vi "BuildTestFromProjectItem_Library_SetsTestSuiteName.vi"() -> ()   [LabVIEW 2017, in "LVUnitTestBuilderTest.lvlib"]
uses:
  LVUnitTestBuilderTest.lvlib
  LVUnitTestBuilder/LVUnitTestBuilder.lvclass
  TestSuite/TestSuite.lvclass
  a12a2084-e44a-4edc-a973-f21fdd0e5ac6.vi
panel:
  out "error out":errorcluster
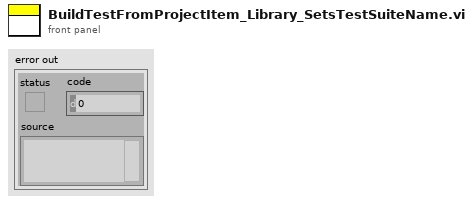
[diagram p1: front panel]
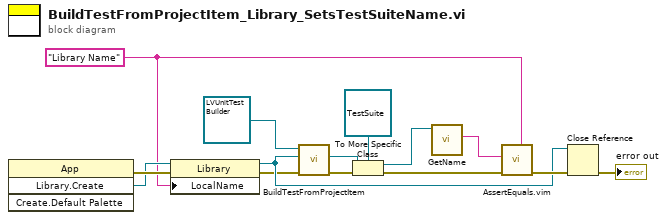
[diagram p0: block diagram]
diagram:
  w1 = "Library Name" ("Localized Name")
  n1 = invoke class="App" method="Library.Create"() -> (error out=w5:errorcluster, "Create Library"=w4:refnum<vi>)  [unwired: 4 in, 2 out]
  n2 = property class="Library"(reference=w4, error in=w5, "LocalName"=w1) -> (reference out=w3:refnum<vi>, error out=w2:errorcluster)
  n3 = call-dynamic "BuildTestFromProjectItem.vi"("error in (no error)"=w2, "ProjectItem Refnum"=w3, "LVUnitTestBuilder in"=refnum<class "LVUnitTestBuilder.lvclass"> refnum ("LVUnitTestBuilder")) -> ("error out"=w9:errorcluster, "Test"=w13:refnum<class "Test.lvclass">)  [unwired: 6 in, 1 out]
  n4 = To More Specific Class(target class=refnum<class "TestSuite.lvclass"> refnum ("TestSuite.lvclass"), reference=w13, error in=w9) -> (specific class reference=w11:refnum<class "TestSuite.lvclass">, error out=w8:errorcluster)
  n5 = call-dynamic "GetName.vi"("TestSuite in"=w11) -> ("Name"=w6:string)  [unwired: 8 in, 2 out]
  n6 = call "AssertEquals.vim"("Expected"=w1, "error in (no error)"=w8, "Actual"=w6) -> ("error out"=w7:errorcluster)  [unwired: 8 in]
  n7 = Close Reference(reference=w3, error in (no error)=w7) -> (error out=→"error out":errorcluster)
